vi "Y.vi"(1 "T":dbl, 2 "V":dbl, 3 "Y(0)":dbl) -> (0 "Y":dbl)   [LabVIEW 2012]
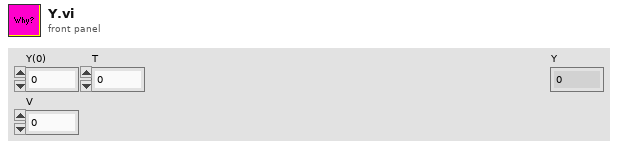
[diagram p1: front panel]
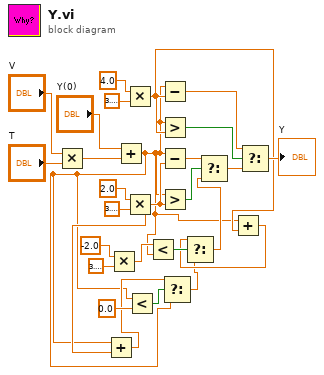
[diagram p0: block diagram]
diagram:
  n1 = Multiply(x="V", y="T") -> (x*y=w25:dbl)
  n2 = Multiply(x=-2.0, y=3.141592653589793) -> (x*y=w9:dbl)
  n3 = Add(x="Y(0)", y=w25) -> (x+y=w1:dbl)
  n4 = Multiply(x=4.0, y=3.141592653589793) -> (x*y=w8:dbl)
  n5 = Multiply(x=2.0, y=3.141592653589793) -> (x*y=w2:dbl)
  n6 = Add(x=w1, y=w2) -> (x+y=w3:dbl)
  n7 = Less?(x=w1, y=0.0) -> (x < y?=w6:bool)
  n8 = Less?(x=w9, y=w1) -> (x < y?=w12:bool)
  n9 = Subtract(x=w1, y=w8) -> (x-y=w20:dbl)
  n10 = Greater?(x=w1, y=w8) -> (0:w21:bool)
  n11 = Subtract(x=w1, y=w2) -> (x-y=w15:dbl)
  n12 = Greater?(x=w1, y=w2) -> (0:w18:bool)
  n13 = Select(t=w3, s=w6, f=w1) -> (s? t:f=w5:dbl)
  n14 = Add(x=w1, y=w8) -> (x+y=w7:dbl)
  n15 = Select(t=w7, s=w12, f=w5) -> (s? t:f=w13:dbl)
  n16 = Select(t=w15, s=w18, f=w13) -> (s? t:f=w19:dbl)
  n17 = Select(t=w20, s=w21, f=w19) -> (s? t:f=→"Y":dbl)
